vi "add img.vi"(7 "error in (no error)":errorcluster caption="Fehler (Eingang, kein Fehler)", 8 "img.lvclass":refnum<class "img.lvclass">, 10 "Segment (Eingang)":refnum<class "Segment.lvclass">) -> (0 "error out":errorcluster caption="Fehler (Ausgang)", 3 "Segment (Ausgang)":refnum<class "Segment.lvclass">)   [LabVIEW 2013, in "DatenKlassen.lvlib" / "Segment.lvclass"]
uses:
  Segment.lvclass
  Image/img.lvclass
  Segment.lvclass/Segment.ctl
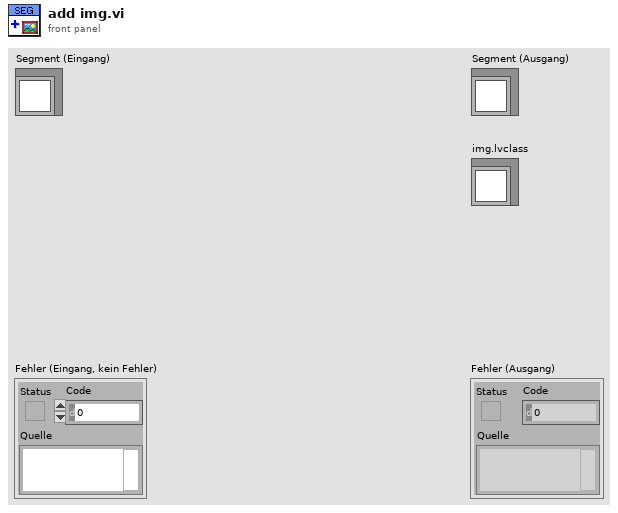
[diagram p1: front panel]
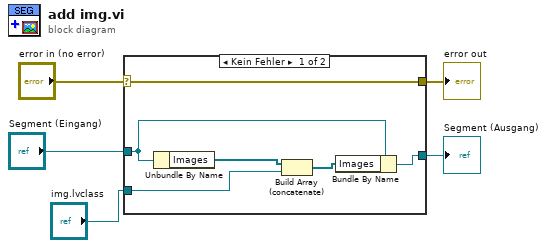
[diagram p0: block diagram]
diagram:
  n1 = case shown="Kein Fehler" "error in (no error)" {
    selector: "error in (no error)" -> [w11 w12]
    tunnel: [w11 w12] -> w4
    tunnel: [w9 w13] -> w2
    tunnel: "Segment (Eingang)" -> [w8 w13]
    tunnel: "img.lvclass" -> [w6 _]
    frame No Error {
      n2 = Unbundle By Name(w8) -> ("Images"=w10:refnum<class "img.lvclass">[])
      n3 = Build Array (concatenate)(w10, w6) -> (w7:refnum<class "img.lvclass">[])
      n4 = Bundle By Name(cluster=w8, "Images"=w7) -> (w9:refnum<class "Segment.lvclass">)
    }
    frame Error {
    }
  }
  "error out" <- w4
  "Segment (Ausgang)" <- w2
